vi "Hex String.vi"(8 "Eingabe String":string) -> (0 "Status":T1)   [LabVIEW 2020, in "Linearisierung v2.lvlib" / "Gasteiler.lvlib" / "Horiba GDC.lvlib"]
uses:
  Horiba GDC.lvlib
  Stats.ctl
panel:
  out "0 Base Gas N2\n1 Base Gas O2":i16
  out "0 Gas Gen Off\n1 Gas Gen On":i16
  out "0 Purge 1 Off\n1 Purge 1 On":i16
  out "0 Purge 2 Off\n1 Purge 2 On":i16
  out "0 Manual Off\n1 Manual On":i16
  out "0 GD not inst\n1 GD installed":i16
  out "0 CC not inst\n1 Cc installed":i16
  out "0 Zero Gas Off\n1 Zero Gas On":i16
  out "0 Span Gas off\n1 Span Gas On":i16
  out "0 O2 Off\n1 O2 On":i16
  out "0 Ozon Off\n1 Ozon On":i16
  out "0 CC\n1 GD":i16
  out "0 local\n1 Remote":i16
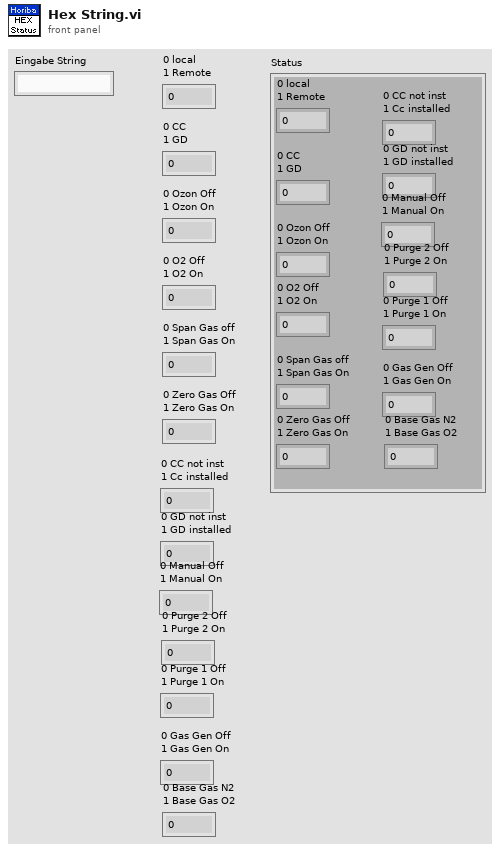
[diagram p1: front panel]
types:
  T1 = typedef "Linearisierung v2.lvlib/Gasteiler.lvlib/Horiba GDC.lvlib/Stats.ctl" = cluster{"0 local\n1 Remote":i16, "0 CC\n1 GD":i16, "0 Ozon Off\n1 Ozon On":i16, "0 O2 Off\n1 O2 On":i16, "0 Span Gas off\n1 Span Gas On ":i16, "0 Zero Gas Off\n1 Zero Gas On":i16, "0 CC not inst\n1 Cc installed":i16, "0 GD not inst\n1 GD installed":i16, "0 Manual Off\n1 Manual On":i16, "0 Purge 2 Off\n1 Purge 2 On":i16, "0 Purge 1 Off\n1 Purge 1 On":i16, "0 Gas Gen Off\n1 Gas Gen On":i16, "0 Base Gas N2\n1 Base Gas O2":i16}
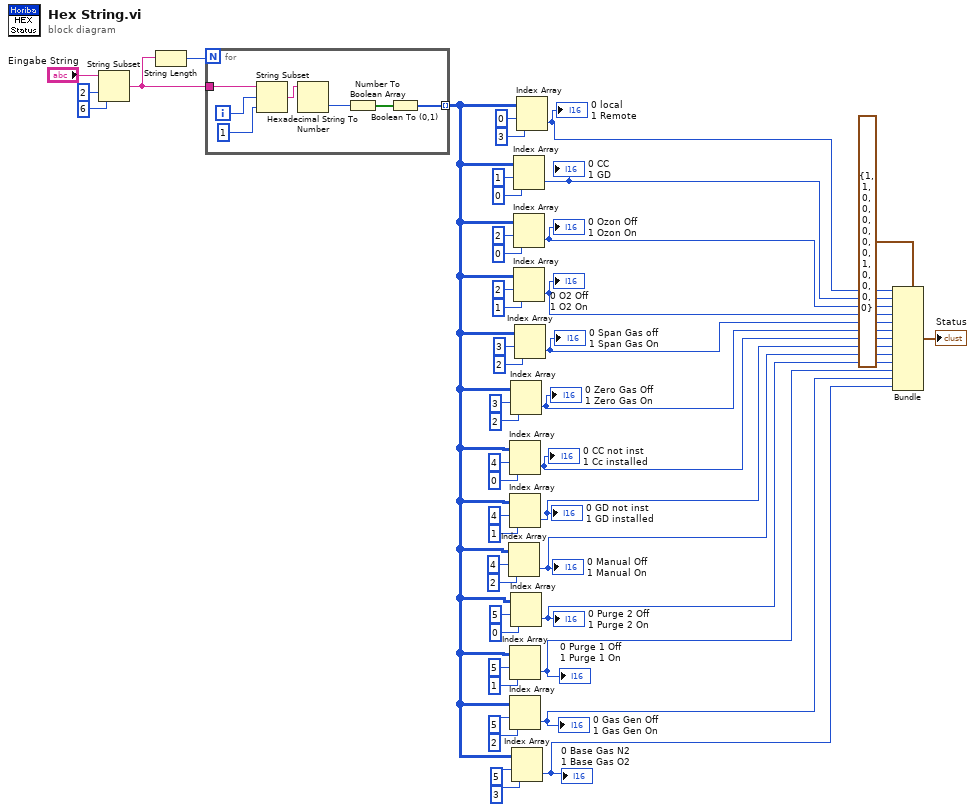
[diagram p0: block diagram]
diagram:
  n1 = String Subset(string="Eingabe String", offset (0)=2 ("Offset (0)"), length (rest)=6 ("Länge (Rest)")) -> (substring=w43:string)
  n2 = String Length(string=w43) -> (length=w44:i32)
  n3 = for {
    N: w44 -> [_]
    tunnel: w43 -> [w54]
    tunnel: [w49] -> w16 mode=indexing
    i -> [w52]
    n4 = String Subset(string=w54, offset (0)=w52, length (rest)=1 ("Länge (Rest)")) -> (substring=w53:string)
    n5 = Hexadecimal String To Number(string=w53) -> (number=w50:u32)  [unwired: 2 in, 1 out]
    n6 = Number To Boolean Array(number=w50) -> (Boolean array=w48:bool[])
    n7 = Boolean To (0,1)(Boolean=w48) -> (0, 1=w49:i16[])
  }
  n8 = Index Array(array=w16, index (row)=4 ("Index (Zeile)"), index (col)=2 ("Deaktivierter Index (Spalte)")) -> (element=w5:i16)
  "0 Manual Off\n1 Manual On" <- w5
  n9 = Index Array(array=w16, index (row)=4 ("Index (Zeile)"), index (col)=0 ("Deaktivierter Index (Spalte)")) -> (element=w7:i16)
  "0 CC not inst\n1 Cc installed" <- w7
  n10 = Index Array(array=w16, index (row)=4 ("Index (Zeile)"), index (col)=1 ("Deaktivierter Index (Spalte)")) -> (element=w6:i16)
  "0 GD not inst\n1 GD installed" <- w6
  n11 = Index Array(array=w16, index (row)=5 ("Index (Zeile)"), index (col)=1 ("Deaktivierter Index (Spalte)")) -> (element=w3:i16)
  "0 Purge 1 Off\n1 Purge 1 On" <- w3
  n12 = Index Array(array=w16, index (row)=5 ("Index (Zeile)"), index (col)=2 ("Deaktivierter Index (Spalte)")) -> (element=w2:i16)
  "0 Gas Gen Off\n1 Gas Gen On" <- w2
  n13 = Index Array(array=w16, index (row)=3 ("Index (Zeile)"), index (col)=2 ("Deaktivierter Index (Spalte)")) -> (element=w8:i16)
  "0 Zero Gas Off\n1 Zero Gas On" <- w8
  n14 = Index Array(array=w16, index (row)=5 ("Index (Zeile)"), index (col)=0 ("Deaktivierter Index (Spalte)")) -> (element=w4:i16)
  "0 Purge 2 Off\n1 Purge 2 On" <- w4
  n15 = Index Array(array=w16, index (row)=5 ("Index (Zeile)"), index (col)=3 ("Deaktivierter Index (Spalte)")) -> (element=w1:i16)
  "0 Base Gas N2\n1 Base Gas O2" <- w1
  n16 = Index Array(array=w16, index (row)=1 ("Index (Zeile)"), index (col)=0 ("Deaktivierter Index (Spalte)")) -> (element=w12:i16)
  "0 CC\n1 GD" <- w12
  n17 = Index Array(array=w16, index (row)=2 ("Index (Zeile)"), index (col)=0 ("Deaktivierter Index (Spalte)")) -> (element=w11:i16)
  "0 Ozon Off\n1 Ozon On" <- w11
  n18 = Index Array(array=w16, index (row)=2 ("Index (Zeile)"), index (col)=1 ("Deaktivierter Index (Spalte)")) -> (element=w10:i16)
  "0 O2 Off\n1 O2 On" <- w10
  n19 = Index Array(array=w16, index (row)=3 ("Index (Zeile)"), index (col)=2 ("Deaktivierter Index (Spalte)")) -> (element=w9:i16)
  "0 Span Gas off\n1 Span Gas On" <- w9
  n20 = Index Array(array=w16, index (row)=0 ("Index (Zeile)"), index (col)=3 ("Deaktivierter Index (Spalte)")) -> (element=w13:i16)
  "0 local\n1 Remote" <- w13
  n21 = Bundle(cluster=T1 {"0 local\n1 Remote"=1, "0 CC\n1 GD"=1, "0 Ozon Off\n1 Ozon On"=0, "0 O2 Off\n1 O2 On"=0, "0 Span Gas off\n1 Span Gas On "=0, "0 Zero Gas Off\n1 Zero Gas On"=0, "0 CC not inst\n1 Cc installed"=0, "0 GD not inst\n1 GD installed"=0, "0 Manual Off\n1 Manual On"=1, "0 Purge 2 Off\n1 Purge 2 On"=0, "0 Purge 1 Off\n1 Purge 1 On"=0, "0 Gas Gen Off\n1 Gas Gen On"=0, "0 Base Gas N2\n1 Base Gas O2"=0} ("Status"), "0 local\n1 Remote"=w13, "0 CC\n1 GD"=w12, "0 Ozon Off\n1 Ozon On"=w11, "0 O2 Off\n1 O2 On"=w10, "0 Span Gas off\n1 Span Gas On"=w9, "0 Zero Gas Off\n1 Zero Gas On"=w8, "0 CC not inst\n1 Cc installed"=w7, "0 GD not inst\n1 GD installed"=w6, "0 Manual Off\n1 Manual On"=w5, "0 Purge 2 Off\n1 Purge 2 On"=w4, "0 Purge 1 Off\n1 Purge 1 On"=w3, "0 Gas Gen Off\n1 Gas Gen On"=w2, "0 Base Gas N2\n1 Base Gas O2"=w1) -> (→"Status":T1)
